vi "Set Active Tree.vi"(8 "error in (no error)":errorcluster, 9 "Tree to set in":refnum<class "Tree.lvclass">, 11 "Tree in":refnum<class "Tree.lvclass">) -> (0 "error out":errorcluster, 1 "Tree set out":refnum<class "Tree.lvclass">, 3 "Tree out":refnum<class "Tree.lvclass">)   [LabVIEW 2015, in "MDSplus.lvlib" / "Tree.lvclass"]
doc: "Set the passed tree as the active one."
uses:
  <vilib>/MDSplus/Classes/Tree_Class/Tree.lvclass
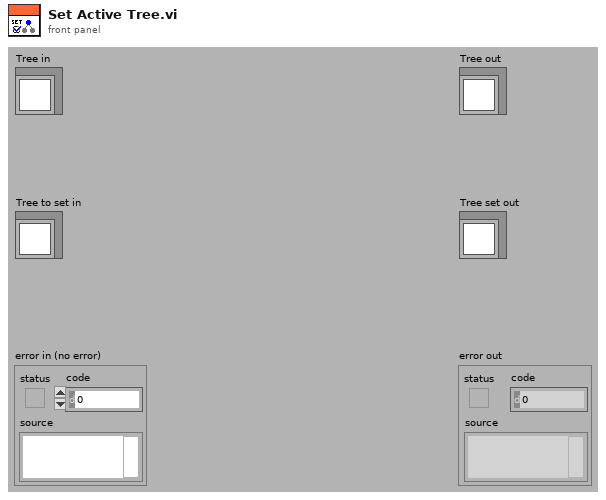
[diagram p1: front panel]
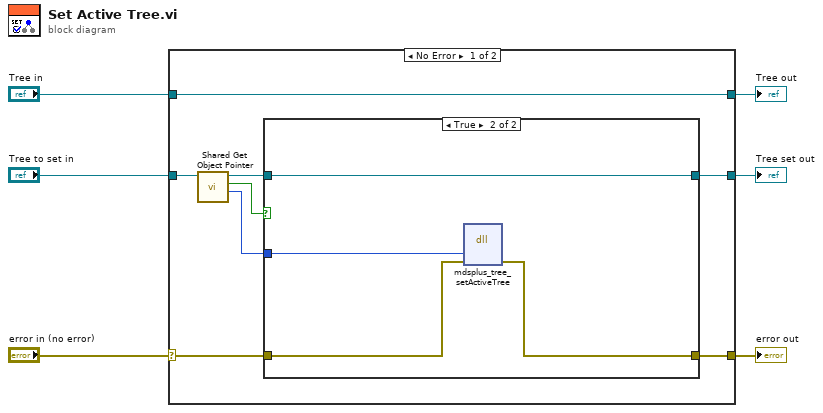
[diagram p0: block diagram]
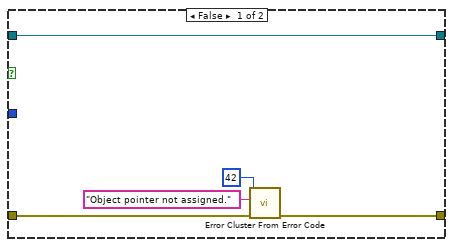
[diagram p2: hidden frame]
diagram:
  n1 = case shown="No Error" "error in (no error)" {
    selector: "error in (no error)" -> [w14 w26]
    tunnel: [w13 w26] -> w5
    tunnel: "Tree to set in" -> [w12 w25]
    tunnel: [w9 w25] -> w4
    tunnel: "Tree in" -> [w7 w24]
    tunnel: [w7 w24] -> w1
    frame No Error {
      n2 = call <vilib>:"Shared Get Object Pointer.vi"("Tree in"=w12) -> ("Object Pointer"=w8:i64, "Assigned object pointer?"=w11:bool, "Tree out"=w10:refnum<class "Tree.lvclass">)  [unwired: 8 in]
      n3 = case shown="True" w11 {
        tunnel: w14 -> [w16 w23]
        tunnel: [w15 w20] -> w13
        tunnel: w10 -> [w19 w22]
        tunnel: [w19 w22] -> w9
        tunnel: w8 -> [_ w21]
        frame False {
          n4 = call <vilib>:"Error Cluster From Error Code.vi"("error in (no error)"=w16, "error message (\"\")"="Object pointer not assigned." ("error message (\"\")"), "error code (0)"=42) -> ("error out"=w15:errorcluster)  [unwired: 6 in]
        }
        frame True {
          n5 = dll-call lib="MDSobjectsLVShr" fn="mdsplus_tree_setActiveTree"("lvTreePtrIn"=w21, "error"=w23) -> ("error"=w20:errorcluster)  [unwired: 5 in, 2 out]
        }
      }
    }
    frame Error {
    }
  }
  "error out" <- w5
  "Tree set out" <- w4
  "Tree out" <- w1
